vi "example 6 - child.vi"() -> ()   [LabVIEW 2020]
panel:
  in  "Invisible - Caption on":bool
  in  "Invisible - Caption off":bool
  in  "Visible - Caption on":bool
  in  "Visible - Caption off":bool
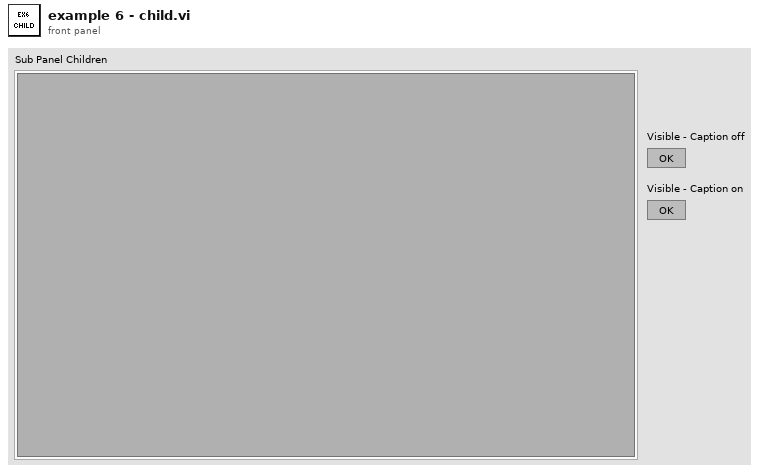
[diagram p1: front panel]
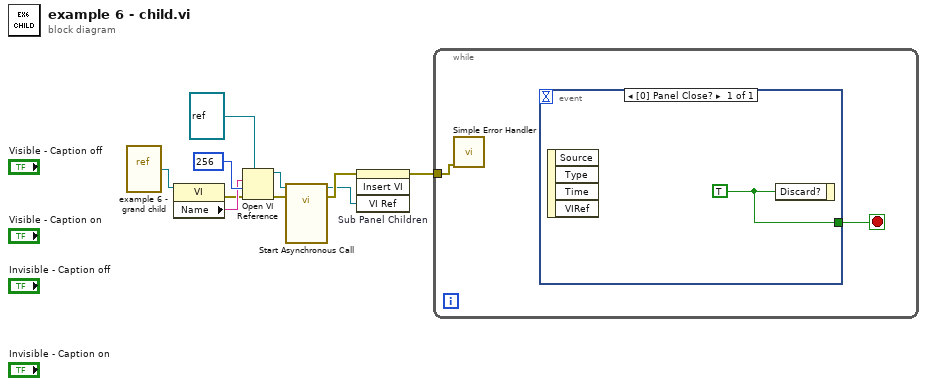
[diagram p0: block diagram]
diagram:
  n1 = vi-ref "example 6 - grand child.vi"() -> (w6:refnum<vi>)
  n2 = property class="VI"(reference=w6) -> (error out=w4:errorcluster, "Name"=w5:string)  [unwired: 1 in, 1 out]
  n3 = Open VI Reference(type specifier VI Refnum (for type only)=refnum<vi> refnum, vi path=w5, options=256 ("call and forget"), error in (no error)=w4) -> (vi reference=w8:refnum<vi>, error out=w7:errorcluster)  [unwired: 2 in]
  n4 = call-by-ref "Start Asynchronous Call"(reference=w8, error in=w7) -> (reference out=w2:refnum<vi>, error out=w3:errorcluster)  [unwired: 12 in]
  n5 = invoke on="Sub Panel Children" class="SubPnl" method="Insert VI"(error in=w3, "VI Ref"=w2) -> (error out=w1:errorcluster)  [unwired: 2 in, 3 out]
  n6 = while {
    tunnel: w1 -> [w11]
    stop <- w12 stop-if-true
    n7 = call <vilib>:"Simple Error Handler.vi"("error in (no error)"=w11) -> ()  [unwired: 4 in, 5 out]
    n8 = event shown="[0] Panel Close?" {
      selector: _ -> [_]
      dyn-events: _ -> [_]
      timeout: _ -> [_]
      tunnel: [w13] -> w12
      event Panel Close? {
        w13 = TRUE
        n9 = event-data() -> ()  [unwired: 1 in, 4 out]
        n10 = event-data("Discard?"=w13) -> ()  [unwired: 1 in, 1 out]
      }
    }
  }
